vi "NetworkTable get.vi"   [LabVIEW 2014]
uses:
  <vilib>/Rock Robotics/Network Tables/SD Read Number.vi
  <vilib>/Rock Robotics/Network Tables/SD Read Boolean.vi
  <vilib>/Rock Robotics/Network Tables/SD Write Number.vi
  <vilib>/Rock Robotics/Network Tables/SD Read String.vi
  Robot Values.vi
  <vilib>/Rock Robotics/Network Tables/SD Write String.vi
types:
  T1 = cluster{"Lift Encoder Height Right (cm)":dbl, "Lift Encoder Height Left (cm)":dbl, "Right Prox":bool, "Left Prox":bool, "Gyro Angle":dbl, "Gyro anglar rate":dbl, "Gyro Reset":bool, "Drive encoder Dash reset":bool}
  T2 = cluster{"DriveMode":enum16{"Tank", "Arcade"}, "Is Logitech":bool}
  T3 = cluster{"Lift Position":i32, "Lift Speed Override":dbl, "OverrideTele?":bool, "OverrideDash":bool}
  T4 = cluster{"Tracking Tote?":bool, "ToteRightSpeed":dbl, "ToteLeftSpeed":dbl, "Drive Encoder reset":bool, "Right Wheel \n(Cm)":dbl, "Left Wheel \n(Cm)":dbl}
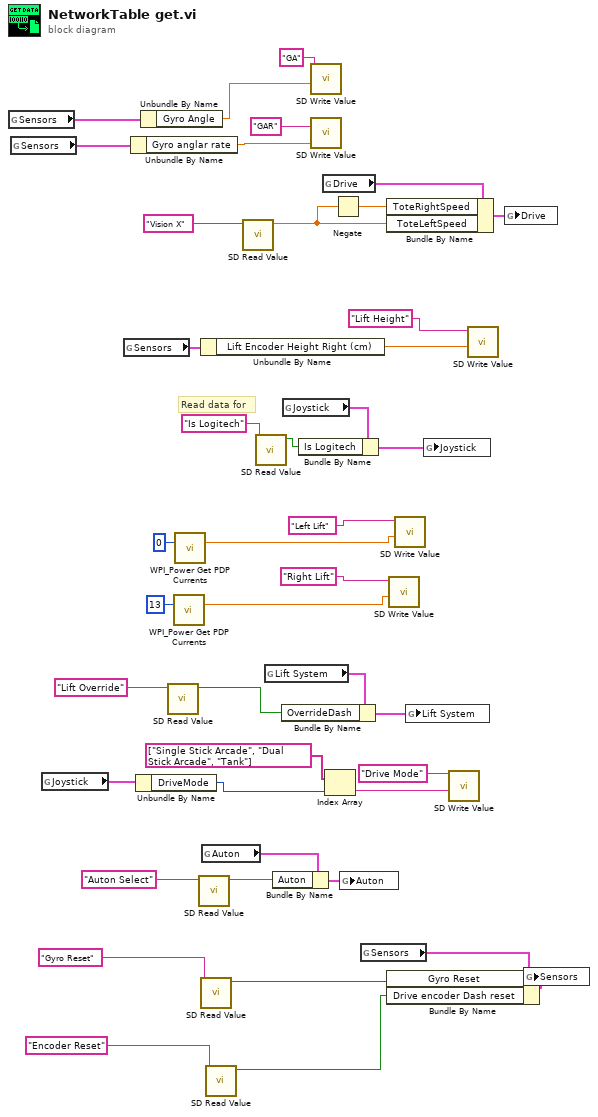
[diagram p0: block diagram]
diagram:
  # "Read data for"
  n1 = global read "Robot Values.vi" "Sensors"() -> (w21:T1)
  n2 = global read "Robot Values.vi" "Sensors"() -> (w20:T1)
  n3 = global read "Robot Values.vi" "Joystick"() -> (w15:T2)
  n4 = global read "Robot Values.vi" "Sensors"() -> (w38:T1)
  n5 = Unbundle By Name(w20) -> ("Gyro anglar rate"=w18:dbl)
  n6 = Unbundle By Name(w15) -> ("DriveMode"=w14:enum16{"Tank", "Arcade"})
  n7 = Unbundle By Name(w21) -> ("Gyro Angle"=w19:dbl)
  n8 = call-poly <vilib>:"SD Read Value.vi"("Name"="Lift Override") -> ("Boolean"=w29:bool)  [unwired: 8 in, 2 out]
  n9 = call <vilib>:"WPI_Power Get PDP Currents.vi"("PDP Channel"=13) -> ("current (A)"=w26:dbl)  [unwired: 12 in, 2 out]
  n10 = call <vilib>:"WPI_Power Get PDP Currents.vi"("PDP Channel"=0) -> ("current (A)"=w24:dbl)  [unwired: 12 in, 2 out]
  n11 = call-poly <vilib>:"SD Read Value.vi"("Name"="Auton Select") -> ("String"=w8:string)  [unwired: 8 in, 2 out]
  n12 = Unbundle By Name(w38) -> ("Lift Encoder Height Right (cm)"=w22:dbl)
  n13 = call-poly <vilib>:"SD Read Value.vi"("Name"="Gyro Reset") -> ("Boolean"=w4:bool)  [unwired: 8 in, 2 out]
  n14 = global read "Robot Values.vi" "Auton"() -> (w9:cluster{"Auton":string})
  n15 = call-poly <vilib>:"SD Read Value.vi"("Name"="Encoder Reset") -> ("Boolean"=w1:bool)  [unwired: 8 in, 2 out]
  n16 = call-poly <vilib>:"SD Read Value.vi"("Name"="Vision X") -> ("Numeric"=w39:dbl)  [unwired: 8 in, 2 out]
  n17 = call-poly <vilib>:"SD Read Value.vi"("Name"="Is Logitech") -> ("Boolean"=w35:bool)  [unwired: 8 in, 2 out]
  n18 = global read "Robot Values.vi" "Lift System"() -> (w31:T3)
  n19 = Bundle By Name(cluster=w9, "Auton"=w8) -> (w7:cluster{"Auton":string})
  n20 = Bundle By Name(cluster=w31, "OverrideDash"=w29) -> (w30:T3)
  n21 = global read "Robot Values.vi" "Joystick"() -> (w36:T2)
  n22 = Bundle By Name(cluster=w36, "Is Logitech"=w35) -> (w34:T2)
  n23 = call-poly <vilib>:"SD Write Value.vi"("Numeric"=w19, "Name"="GA") -> ()  [unwired: 8 in, 2 out]
  n24 = call-poly <vilib>:"SD Write Value.vi"("Numeric"=w18, "Name"="GAR") -> ()  [unwired: 8 in, 2 out]
  n25 = global read "Robot Values.vi" "Drive"() -> (w41:T4)
  n26 = Index Array(array=string[] ["Single Stick Arcade", "Dual Stick Arcade", "Tank"], index=w14) -> (element=w12:string)
  n27 = Negate(x=w39) -> (-x=w40:dbl)
  n28 = global write "Robot Values.vi" "Auton"(w7) -> ()
  n29 = global read "Robot Values.vi" "Sensors"() -> (w6:T1)
  n30 = Bundle By Name(cluster=w41, "ToteRightSpeed"=w40, "ToteLeftSpeed"=w39) -> (w42:T4)
  n31 = Bundle By Name(cluster=w6, "Gyro Reset"=w4, "Drive encoder Dash reset"=w1) -> (w5:T1)
  n32 = call-poly <vilib>:"SD Write Value.vi"("Numeric"=w26, "Name"="Right Lift") -> ()  [unwired: 8 in, 2 out]
  n33 = call-poly <vilib>:"SD Write Value.vi"("Numeric"=w24, "Name"="Left Lift") -> ()  [unwired: 8 in, 2 out]
  n34 = global write "Robot Values.vi" "Lift System"(w30) -> ()
  n35 = global write "Robot Values.vi" "Joystick"(w34) -> ()
  n36 = call-poly <vilib>:"SD Write Value.vi"("String"=w12, "Name"="Drive Mode") -> ()  [unwired: 8 in, 2 out]
  n37 = call-poly <vilib>:"SD Write Value.vi"("Numeric"=w22, "Name"="Lift Height") -> ()  [unwired: 8 in, 2 out]
  n38 = global write "Robot Values.vi" "Drive"(w42) -> ()
  n39 = global write "Robot Values.vi" "Sensors"(w5) -> ()
